vi "EXDIR-YAML_DetermineSubdictionaryLength.vi"(10 "start":i32, 11 "ENTIRE Array of YAML Lines":string[](array[string])) -> (2 "indent size of this subdictionary":i32, 3 "Length":i32)   [LabVIEW 2016]
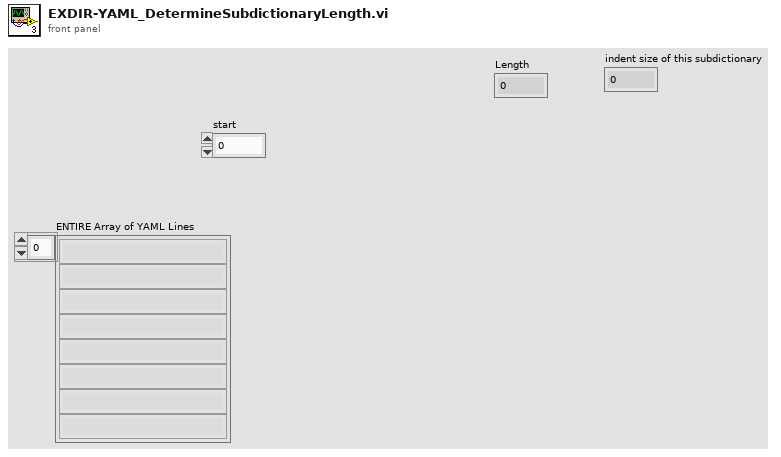
[diagram p1: front panel]
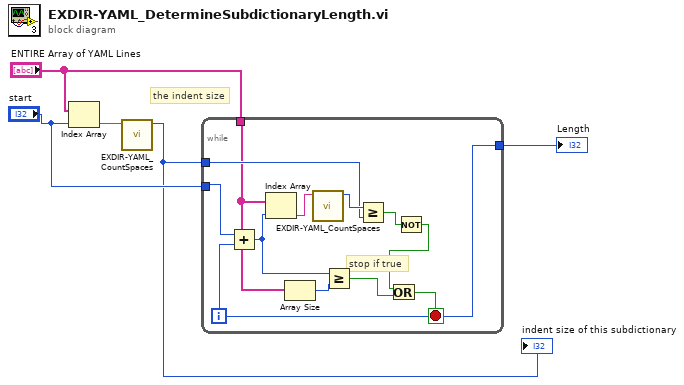
[diagram p0: block diagram]
diagram:
  # "the indent size"
  n1 = Index Array(array="ENTIRE Array of YAML Lines", index="start") -> (element=w5:string)
  n2 = call "EXDIR-YAML_CountSpaces.vi"("String"=w5) -> ("Numeric"=w2:i32)  [unwired: 10 in]
  "indent size of this subdictionary" <- w2
  n3 = while {
    tunnel: "ENTIRE Array of YAML Lines" -> [w13]
    tunnel: "start" -> [w17]
    tunnel: w2 -> [w14]
    tunnel: [w6] -> w1
    i -> [w6]
    stop <- w7 stop-if-true
    # "stop if true"
    n4 = Add(x=w17, y=w6) -> (x+y=w11:i32)
    n5 = Index Array(array=w13, index=w11) -> (element=w16:string)
    n6 = Array Size(array=w13) -> (size(s)=w12:i32)
    n7 = call "EXDIR-YAML_CountSpaces.vi"("String"=w16) -> ("Numeric"=w15:i32)  [unwired: 10 in]
    n8 = Greater Or Equal?(x=w11, y=w12) -> (x >= y?=w9:bool)
    n9 = Greater Or Equal?(x=w15, y=w14) -> (x >= y?=w10:bool)
    n10 = Not(x=w10) -> (.not. x?=w8:bool)
    n11 = Or(x=w8, y=w9) -> (x .or. y?=w7:bool)
  }
  "Length" <- w1
